vi "IMUSafety(SubVI).vi"(8 "error in (no error)":errorcluster, 11 "PigeonIMUDevRef":T1 {"Type" items=["CAN"=352321536, "TalonSRX"=33554432]}) -> (3 "Boolean":bool)   [LabVIEW 2019]
uses:
  <vilib>/Rock Robotics/WPI/ThirdParty/Phoenix-LabVIEW/Pigeon IMU/CTRE_PigeonIMU_GetTempStateUpTime.vi
  <vilib>/Rock Robotics/WPI/ThirdParty/Phoenix-LabVIEW/Pigeon IMU/CTRE_PigeonIMU_ConnectionType.ctl
  <vilib>/Rock Robotics/WPI/ThirdParty/Phoenix-LabVIEW/Pigeon IMU/CTRE_PigeonIMU_DeviceRef.ctl
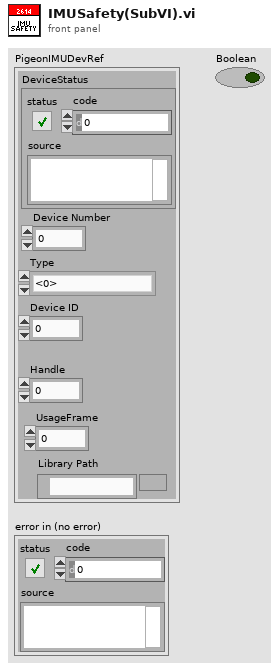
[diagram p1: front panel]
types:
  T1 = typedef "CTRE_PigeonIMU_DeviceRef.ctl" = cluster{"DeviceStatus":errorcluster, "Device Number":u8, "Type":T2, "Device ID":u32, "Handle":u64, "UsageFrame":u32, "Library Path":path}
  T2 = typedef "CTRE_PigeonIMU_ConnectionType.ctl" = u32
  T3 = typedef "CTRE_PigeonIMU_CalibrationMode.ctl" = u16
  T4 = typedef "CTRE_PigeonIMU_PigeonState.ctl" = enum16{"NoComm", "Initializing", "Ready", "UserCalibration"}
  T5 = cluster{"CurrentMode":T3, "LastCalError":i32, "CalBooting?":bool, "PigeonState":T4, "UpTime":u32, "Temp. (C)":dbl, "Temp Compensation Event Count":u32, "No Motion Event Count":u32}
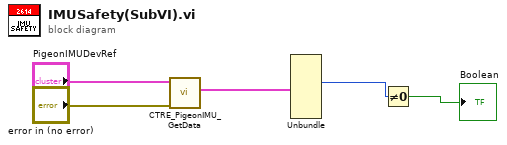
[diagram p0: block diagram]
diagram:
  n1 = call-poly <vilib>:"CTRE_PigeonIMU_GetData.vi"("error in (no error)"="error in (no error)", "PigeonIMUDevRef"="PigeonIMUDevRef") -> ("Temp/State/UpTime"=w1:T5)  [unwired: 7 in, 2 out]
  n2 = Unbundle(w1) -> ("PigeonState"=w4:T4)  [unwired: 7 out]
  n3 = Not Equal To 0?(x=w4) -> (x != 0?=→"Boolean":bool)
